vi "Transceiver Thread.Initialize.vi"(8 "error in (no error)":errorcluster, 11 "Transceiver Thread in":refnum<class "Transceiver Thread.lvclass">) -> (0 "error out":errorcluster, 3 "Transceiver Thread out":refnum<class "Transceiver Thread.lvclass">)   [LabVIEW 2017, in "DSF Core.lvlib" / "Transceiver Thread.lvclass"]
uses:
  Transceiver Thread.lvclass
  Transceiver Thread.lvclass/Transceiver Thread.ctl
  Transfer/Transfer Group.lvclass
  Transceiver.lvclass
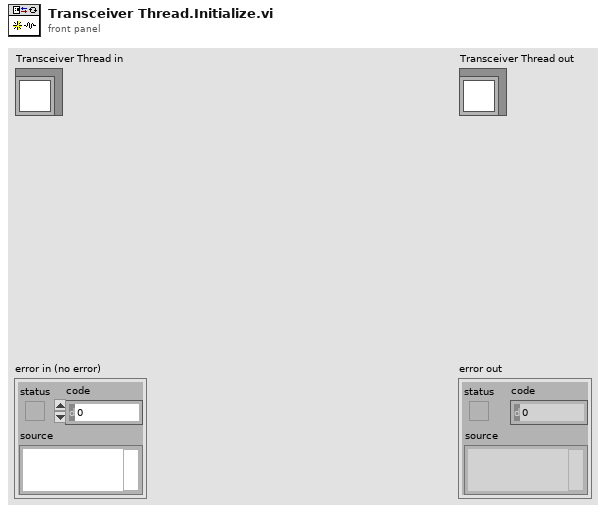
[diagram p1: front panel]
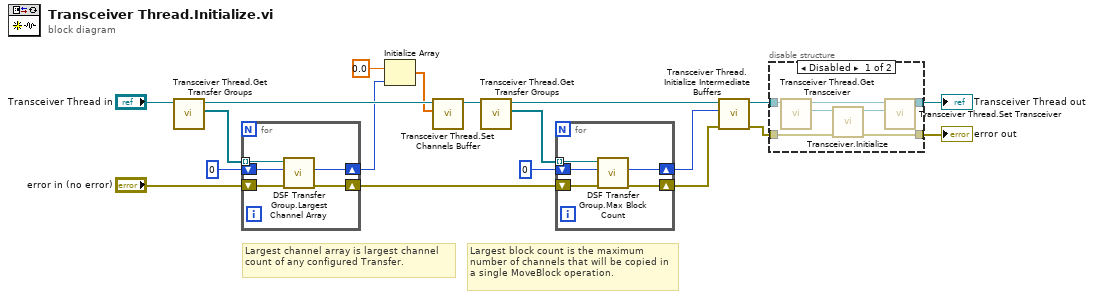
[diagram p0: block diagram]
diagram:
  # "Largest channel array is largest channel count of any configured Transfer."
  # "Largest block count is the maximum number of channels that will be copied in a single MoveBlock operation."
  n1 = call "Transceiver Thread.Get Transfer Groups.vi"("Transceiver Thread in"="Transceiver Thread in") -> ("Transfer Groups"=w8:refnum<class "Transfer Group.lvclass">[], "Transceiver Thread out"=w16:refnum<class "Transceiver Thread.lvclass">)  [unwired: 9 in]
  n2 = for {
    tunnel: w8 -> [w24] mode=indexing
    shift-right: [w20] -> w7
    shift-left: u64 0 ("max channel count") -> [w23]
    shift-right: [w21] -> w4
    shift-left: "error in (no error)" -> [w22]
    n3 = call "DSF Transfer Group.Largest Channel Array.vi"("error in (no error)"=w22, "largest channel array in (0)"=w23, "Transfer Group in"=w24) -> ("error out"=w21:errorcluster, "largest channel array out"=w20:u64)  [unwired: 6 in, 1 out]
  }
  n4 = Initialize Array(0.0 ("element"), w7) -> (w15:dbl[])
  n5 = call "Transceiver Thread.Set Channels Buffer.vi"("channels buffer"=w15, "Transceiver Thread in"=w16) -> ("Transceiver Thread out"=w14:refnum<class "Transceiver Thread.lvclass">)  [unwired: 9 in]
  n6 = call "Transceiver Thread.Get Transfer Groups.vi"("Transceiver Thread in"=w14) -> ("Transfer Groups"=w1:refnum<class "Transfer Group.lvclass">[], "Transceiver Thread out"=w13:refnum<class "Transceiver Thread.lvclass">)  [unwired: 9 in]
  n7 = for {
    tunnel: w1 -> [w29] mode=indexing
    shift-right: [w25] -> w2
    shift-left: u64 0 ("max channel count") -> [w28]
    shift-right: [w26] -> w3
    shift-left: w4 -> [w27]
    n8 = call "DSF Transfer Group.Max Block Count.vi"("error in (no error)"=w27, "previous block count (0)"=w28, "Transfer Group in"=w29) -> ("error out"=w26:errorcluster, "largest block count"=w25:u64)  [unwired: 6 in, 1 out]
  }
  n9 = call "Transceiver Thread.Initialize Intermediate Buffers.vi"("error in (no error)"=w3, "largest block count"=w2, "Transceiver Thread in"=w13) -> ("error out"=w10:errorcluster, "Transceiver Thread out"=w11:refnum<class "Transceiver Thread.lvclass">)  [unwired: 7 in]
  n10 = disable-structure shown="Disabled" {
    disable-tunnel: [w33 w37] -> w19
    disable-tunnel: [w32 w38] -> w18
    disable-tunnel: w11 -> [w31 w38]
    disable-tunnel: w10 -> [w30 w37]
    frame Disabled {
      n11 = call "Transceiver Thread.Get Transceiver.vi"("Transceiver Thread in"=w31) -> ("Transceiver"=w36:refnum<class "Transceiver.lvclass">, "Transceiver Thread out"=w34:refnum<class "Transceiver Thread.lvclass">)  [unwired: 9 in]
      n12 = call-dynamic "Transceiver.Initialize.vi"("error in (no error)"=w30, "Transceiver in"=w36) -> ("error out"=w33:errorcluster, "Transceiver out"=w35:refnum<class "Transceiver.lvclass">)  [unwired: 8 in]
      n13 = call "Transceiver Thread.Set Transceiver.vi"("Transceiver"=w35, "Transceiver Thread in"=w34) -> ("Transceiver Thread out"=w32:refnum<class "Transceiver Thread.lvclass">)  [unwired: 9 in]
    }
    frame Enabled {
    }
  }
  "error out" <- w19
  "Transceiver Thread out" <- w18
